vi "Evaluate.vi"(8 "error in (no error)":errorcluster, 11 "One Of In":refnum<class "One.lvclass">) -> (0 "error out":errorcluster, 1 "Message":string, 2 "Passed?":bool)   [LabVIEW 2020, in "One.lvclass"]
uses:
  One.lvclass
  One.lvclass/One.ctl
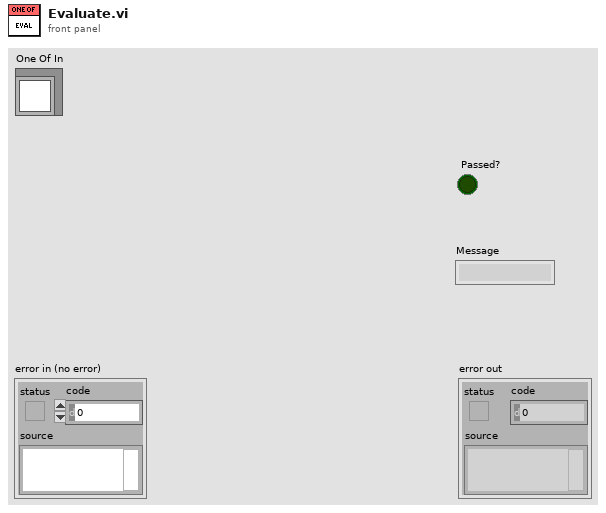
[diagram p1: front panel]
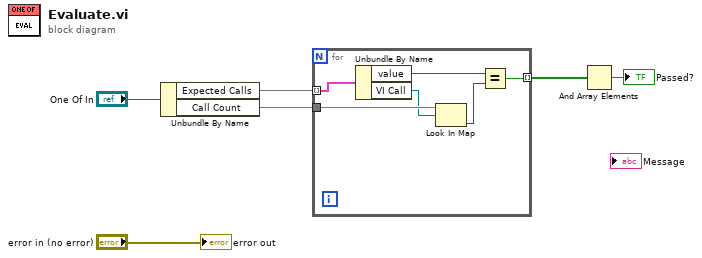
[diagram p0: block diagram]
diagram:
  n1 = Unbundle By Name("One Of In") -> ("Expected Calls"=w4:map{refnum<class "VI Call.lvclass">, i32}, "Call Count"=w3:map{refnum<class "VI Call.lvclass">, i32})
  n2 = for {
    tunnel: w4 -> [w11] mode=indexing
    tunnel: w3 -> [w12]
    tunnel: [w7] -> w2 mode=indexing
    n3 = Unbundle By Name(w11) -> ("value"=w8:i32, "VI Call"=w10:refnum<class "VI Call.lvclass">)
    n4 = Look In Map(map=w12, key=w10) -> (value=w9:i32)  [unwired: 1 in, 1 out]
    n5 = Equal?(x=w8, y=w9) -> (x = y?=w7:bool)
  }
  n6 = And Array Elements(Boolean array=w2) -> (logical AND=→"Passed?":bool)
  "error out" <- "error in (no error)"
